vi "Init Front Panel.vi"(8 "error in":errorcluster, 11 "VI Reference":refnum<vi>) -> (0 "error out":errorcluster)   [LabVIEW 2022 SP3]
doc: "Initialises or sets up the user-facing front panel (GUI) of the application.\nIncludes:\n1. Setting up the area of the front panel that is displayed to the user\n2. Opening or displaying the front panel"
uses:
  <vilib>/Utility/miscctls.llb/LVPointTypeDef.ctl
  <vilib>/Utility/miscctls.llb/LVRectTypeDef.ctl
panel:
  # "Development\ncontrols/indicators useful for development and testing, but which are not outputs of the VI"
  # "Input\nInputs to the VI"
  # "Output\nOutputs of the VI"
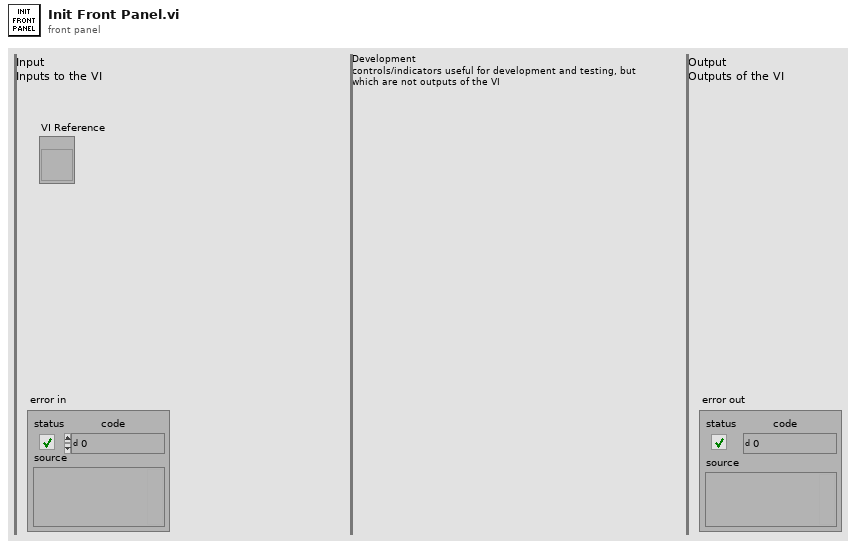
[diagram p1: front panel]
types:
  T1 = enum32{"Invalid", "Standard", "Closed", "Hidden", "Minimized", "Maximized"}
  T2 = typedef "LVRectTypeDef.ctl" = cluster{"Left":i16, "Top":i16, "Right":i16, "Bottom":i16}
  T3 = typedef "LVPointTypeDef.ctl" = cluster{"Horizontal":i16, "Vertical":i16}
  T4 = enum16{"Always On", "Always Off", "Off While Running"}
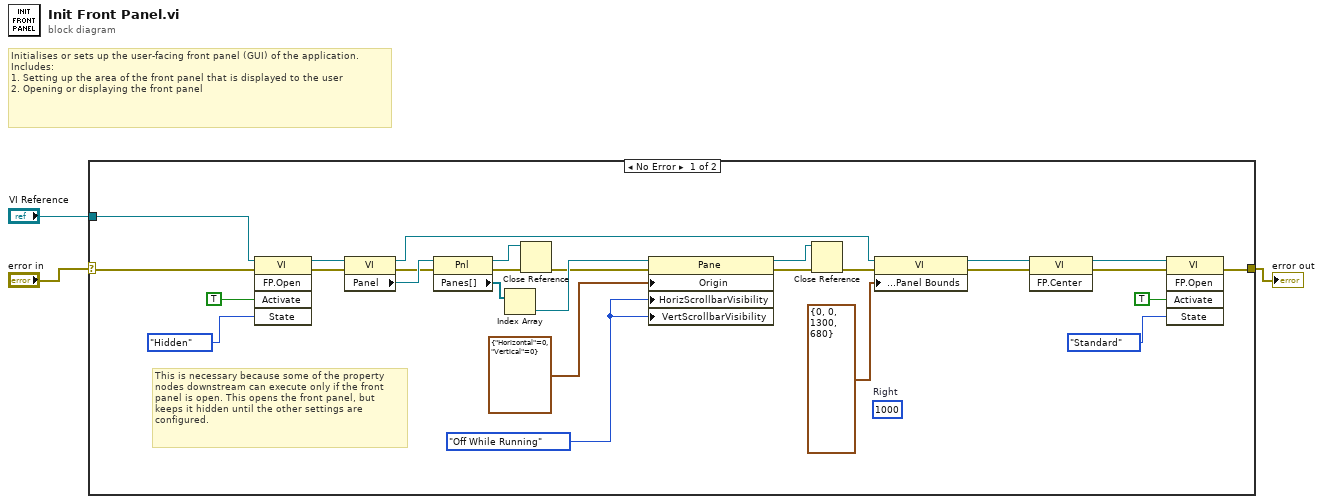
[diagram p0: block diagram]
diagram:
  # "Initialises or sets up the user-facing front panel (GUI) of the application.\nIncludes:\n1. Setting up the area of the front panel that is displayed to the user\n2. Opening or displaying the front panel"
  n1 = case shown="No Error" "error in" {
    selector: "error in" -> [w14 w31]
    tunnel: [w17 w31] -> w2
    tunnel: "VI Reference" -> [w13 _]
    frame No Error {
      (unwired) i16 1000  # Right
      w6 = T4."Off While Running" ("Horizontal Scrollbar Visibility")
      # "This is necessary because some of the property nodes downstream can execute only if the front panel is open. This opens the front panel, but keeps it hidden until the other settings are configured."
      n2 = invoke class="VI" method="FP.Open"(reference=w13, error in=w14, "Activate"=TRUE ("Activate?"), "State"=T1."Hidden") -> (reference out=w11:refnum<vi>, error out=w12:errorcluster)  [unwired: 1 in, 3 out]
      n3 = property class="VI"(reference=w11, error in=w12) -> (reference out=w21:refnum<vi>, error out=w25:errorcluster, "Panel"=w28:refnum<vi>)
      n4 = property class="Pnl"(reference=w28, error in=w25) -> (reference out=w4:refnum<vi>, error out=w24:errorcluster, "Panes[]"=w27:refnum<vi>[])
      n5 = Index Array(array=w27) -> (element=w26:refnum<vi>)  [unwired: 1 in]
      n6 = Close Reference(reference=w4, error in (no error)=w24) -> (error out=w5:errorcluster)
      n7 = property class="Pane"(reference=w26, error in=w5, "Origin"=T3 {"Horizontal"=0, "Vertical"=0}, "HorizScrollbarVisibility"=w6, "VertScrollbarVisibility"=w6) -> (reference out=w19:refnum<vi>, error out=w22:errorcluster)
      n8 = Close Reference(reference=w19, error in (no error)=w22) -> (error out=w20:errorcluster)
      n9 = property on="Property Node" class="VI"(reference=w21, error in=w20, "Front Panel Window:Panel Bounds"=T2 {"Left"=0, "Top"=0, "Right"=1300, "Bottom"=680}) -> (reference out=w10:refnum<vi>, error out=w8:errorcluster)
      n10 = invoke class="VI" method="FP.Center"(reference=w10, error in=w8) -> (reference out=w9:refnum<vi>, error out=w7:errorcluster)  [unwired: 1 in, 1 out]
      n11 = invoke class="VI" method="FP.Open"(reference=w9, error in=w7, "Activate"=TRUE ("Activate?"), "State"=T1."Standard") -> (error out=w17:errorcluster)  [unwired: 1 in, 4 out]
    }
    frame Error {
    }
  }
  "error out" <- w2
